vi "Remove Corners.vi"(3 "Old corners":cluster{"X":dbl, "Y":dbl}[](array[cluster]), 4 "Updated Map":T1) -> (1 "New old corners":cluster{"X":dbl, "Y":dbl}[](array[cluster]))   [LabVIEW 2009]
uses:
  <vilib>/Analysis/Matrix/Datatypes/RealMatrix.ctl
  <vilib>/Analysis/Matrix/NI_Matrix.lvlib
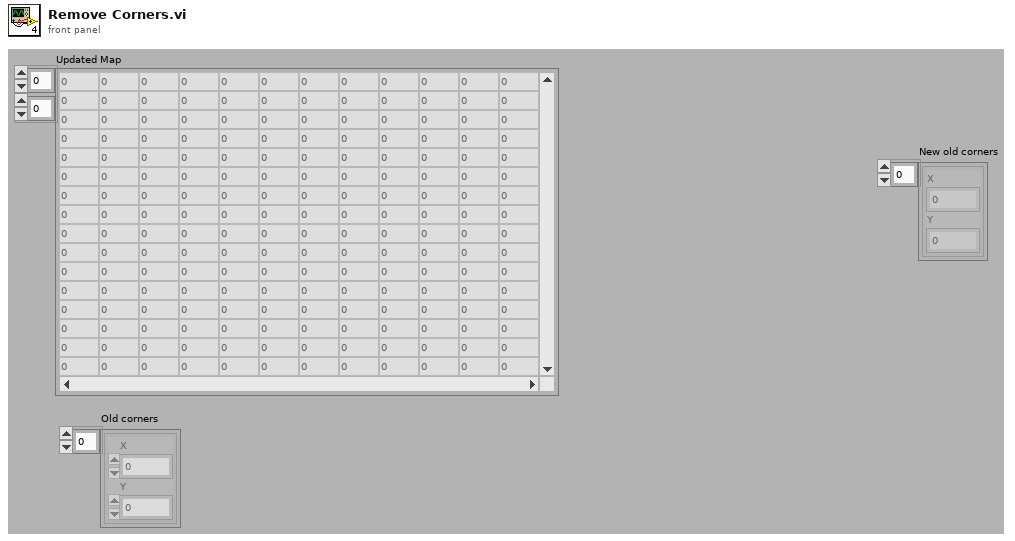
[diagram p1: front panel]
types:
  T1 = typedef "NI_Matrix.lvlib/RealMatrix.ctl" = dbl[][]
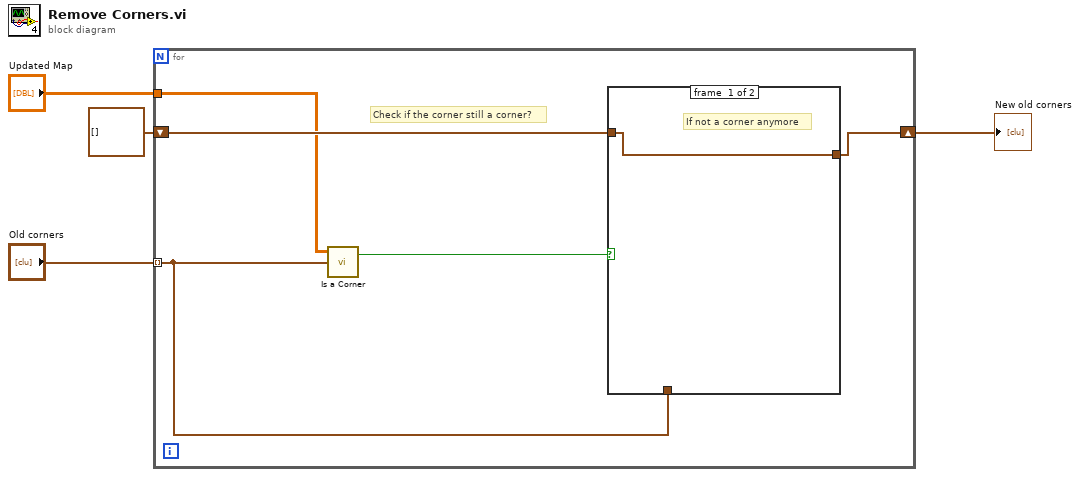
[diagram p0: block diagram]
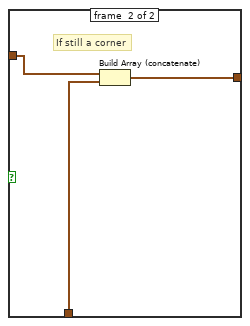
[diagram p2: hidden frame]
diagram:
  n1 = for {
    tunnel: "Old corners" -> [w6] mode=indexing
    tunnel: "Updated Map" -> [w7]
    shift-right: [w8] -> w2
    shift-left: cluster{"X":dbl, "Y":dbl}[] [] -> [w9]
    # "Check if the corner still a corner?"
    n2 = call "Is a Corner.vi"("Corner candidate"=w6, "Updated Map"=w7) -> ("Is a corner"=w5:bool)  [unwired: 2 in]
    n3 = case shown="True" w5 {
      tunnel: w9 -> [w10 w13]
      tunnel: [w10 w12] -> w8
      tunnel: w6 -> [_ w11]
      frame #0 {
        # "If not a corner anymore"
      }
      frame #1 {
        # "If still a corner"
        n4 = Build Array (concatenate)(w13, w11) -> (w12:cluster{"X":dbl, "Y":dbl}[])
      }
    }
  }
  "New old corners" <- w2
